vi "test IO.vi"() -> ()   [LabVIEW 2015]
uses:
  <vilib>/MakerHub/LINX/Public/Peripherals/Digital/Digital Write N Chans.vi
  <vilib>/MakerHub/LINX/Public/Peripherals/Analog/Analog Read N Chans.vi
  <vilib>/MakerHub/LINX/Public/Peripherals/Digital/Digital Read N Chans.vi
  <vilib>/MakerHub/LINX/Private/Local IO/LinxDigitalWrite.vi
  <vilib>/MakerHub/LINX/Public/Utilities/Check Channel.vi
  <vilib>/MakerHub/LINX/Private/Local IO/LinxAnalogRead.vi
  <vilib>/MakerHub/LINX/Private/Local IO/LinxDigitalRead.vi
  <vilib>/MakerHub/LINX/Public/Utilities/Open Serial.vi
  <vilib>/MakerHub/LINX/Private/Utilties/Generate Error.vi
  <vilib>/MakerHub/LINX/LMH-LINX.lvlib
panel:
  in  "Values 2":bool[](array[boolean])
  in  "Frequency (Hz)":u32
  in  "pulse pin":u8
  in  "?":bool
  in  "Serial Port":refnum<visa-resource-name>="N/A"
  out "Waveform Chart":dbl[](graph)
  out "Values":bool[](array[boolean])
  in  "AI Channel(s)":u8[](array[numeric])
  in  "DI Channels":u8[](array[numeric])=[8, 9]
  in  "DO Channels":u8[](array[numeric])
  # "PULSE"
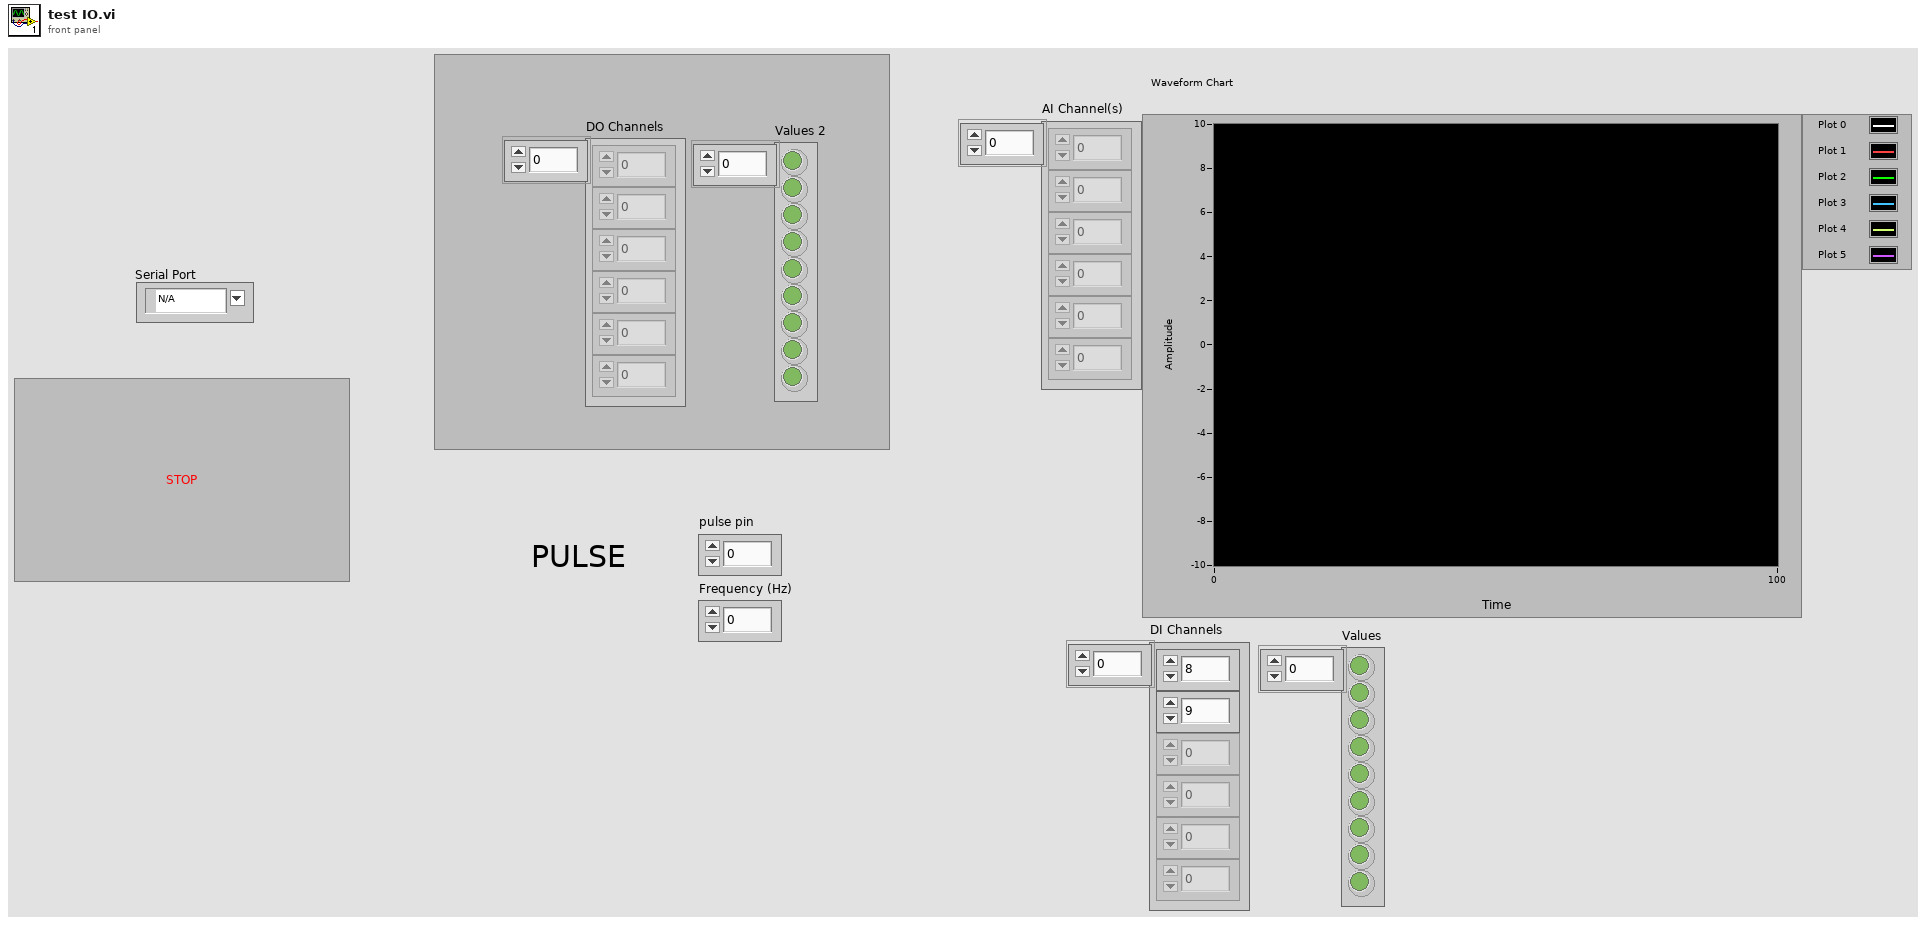
[diagram p1: front panel]
types:
  T1 = typedef "LMH-LINX.lvlib/LINX Ref.ctl" = cluster{"IO":T2, "Interface":T3, "LINX Device Config":T4}
  T2 = typedef "LMH-LINX.lvlib/Platform.ctl" = enum16{"Remote", "Local"}
  T3 = typedef "LMH-LINX.lvlib/Interface.ctl" = enum16{"Serial", "TCP"}
  T4 = typedef "LMH-LINX.lvlib/Device.lvlib/LINX Device Config.ctl" = cluster{"Interface":T3, "COM Port":refnum<visa-resource-name>, "TCP Configuration":T5, "Device Family":u8, "Device ID":u8, "Device Name":string, "TCP Ref":refnum<k5>, "Channels":T6}
  T5 = typedef "LMH-LINX.lvlib/Device.lvlib/TCP Config.ctl" = cluster{"IP Address":string, "Port":u16}
  T6 = typedef "LMH-LINX.lvlib/Channels.ctl" = cluster{"DI":u8[], "DO":u8[], "AI":u8[], "AO":u8[], "PWM":u8[], "QE":u8[], "UART":u8[], "I2C 2":u8[], "SPI":u8[], "CAN":u8[], "Servo":u8[], "AI Ref (V)":dbl, "AI Resolution (Bits)":u8, "AO Ref (V)":dbl, "AO Resolution (Bits)":u8}
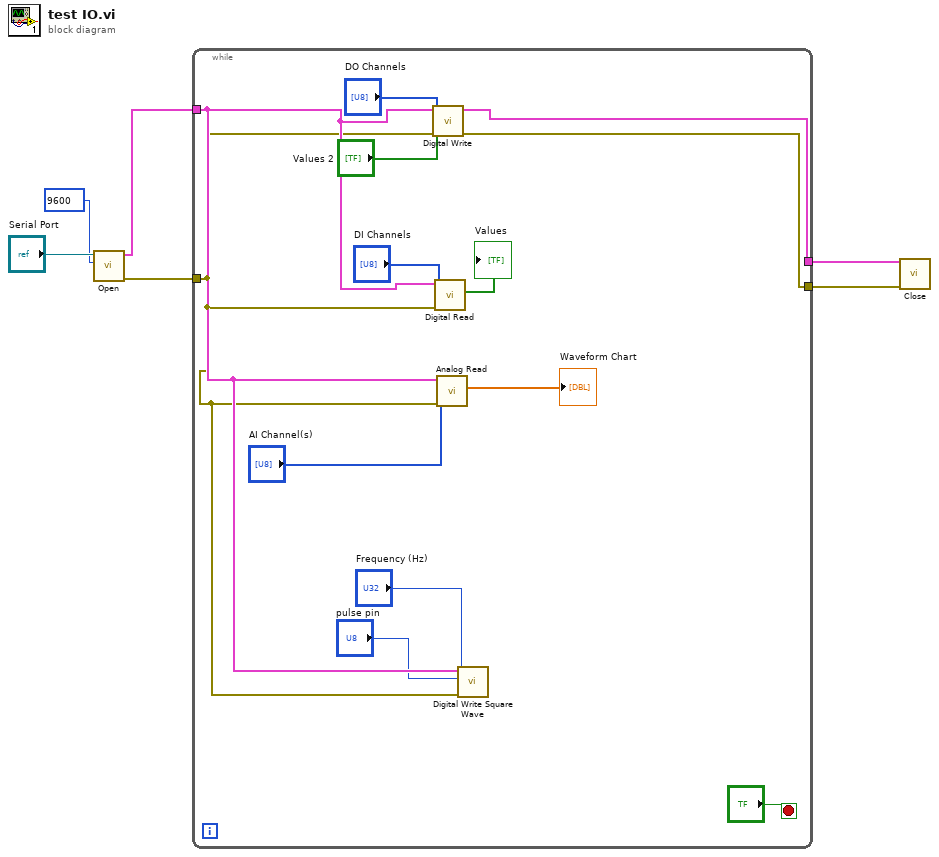
[diagram p0: block diagram]
diagram:
  n1 = call-poly <vilib>:"Open.vi"("Baud Rate Override"=u32 9600, "Serial Port"="Serial Port") -> ("Error Out"=w5:errorcluster, "LINX Resource"=w6:T1)  [unwired: 7 in, 1 out]
  n2 = while {
    tunnel: w6 -> [w11]
    tunnel: w5 -> [w10]
    tunnel: [w15] -> w4
    tunnel: [w14] -> w3
    stop <- "?" stop-if-true
    n3 = call-poly <vilib>:"Digital Write.vi"("Error In"=w10, "Values"="Values 2", "DO Channels"="DO Channels", "LINX Resource"=w11) -> ("Error Out"=w14:errorcluster, "LINX Resource"=w15:T1)  [unwired: 6 in]
    n4 = call-poly <vilib>:"Digital Read.vi"("Error In"=w10, "DI Channels"="DI Channels", "LINX Resource"=w11) -> ("Values"=→"Values":bool[])  [unwired: 6 in, 2 out]
    n5 = call-poly <vilib>:"Analog Read.vi"("Error In"=w10, "AI Channel(s)"="AI Channel(s)", "LINX Resource"=w11) -> ("Voltages"=→"Waveform Chart":dbl[])  [unwired: 5 in, 3 out]
    n6 = call <vilib>:"Digital Write Square Wave.vi"("Error In"=w10, "Frequency (Hz)"="Frequency (Hz)", "Channel"="pulse pin", "LINX Resource"=w11) -> ()  [unwired: 6 in, 2 out]
  }
  n7 = call <vilib>:"Close.vi"("Error In"=w3, "LINX Resource"=w4) -> ()  [unwired: 9 in, 1 out]
